vi "Init.vi"(7 "I2C #":T1=-1, 8 "error in (no error)":errorcluster, 10 "Session In":refnum<class "Session.lvclass">) -> (0 "error out":errorcluster, 3 "Grove Temperature Humidity Sensor DH20 Out":refnum<class "Grove Temperature Humidity Sensor DH20.lvclass">)   [LabVIEW 2020, in "CTI-Peripheral.lvlib" / "Grove Temperature Humidity Sensor DH20.lvclass"]
uses:
  Grove Temperature Humidity Sensor DH20.lvclass
  CTI/Session/Session.lvclass
  CTI/I2C Number.ctl
  CTI/I2C Address.ctl
  CTI/I2C Connection/I2C Connection.lvclass/I2C Connection.ctl
  Grove Temperature Humidity Sensor DH20.lvclass/Grove Temperature Humidity Sensor DH20.ctl
  CTI/I2C Connection/I2C Connection.lvclass
  CTI/CTI.lvlib
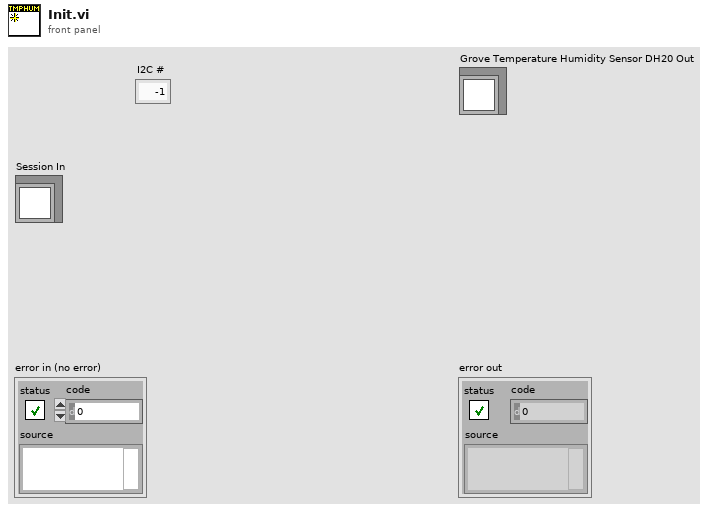
[diagram p1: front panel]
types:
  T1 = typedef "CTI.lvlib/I2C Number.ctl" = i8
  T2 = typedef "CTI.lvlib/I2C Address.ctl" = u8
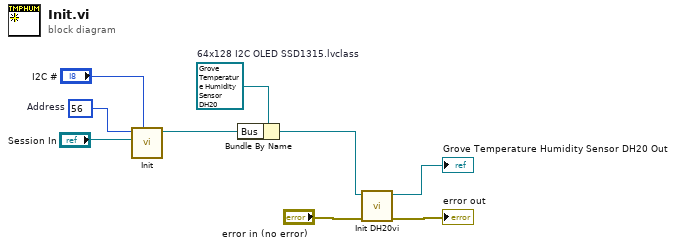
[diagram p0: block diagram]
diagram:
  w5 = refnum<class "Grove Temperature Humidity Sensor DH20.lvclass"> refnum  # 64x128 I2C OLED SSD1315.lvclass
  w6 = T2 56  # Address
  n1 = call "Init.vi"("I2C #"="I2C #", "Session"="Session In", "Address"=w6) -> ("I2C Connection"=w9:refnum<class "I2C Connection.lvclass">)  [unwired: 7 in, 1 out]
  n2 = Bundle By Name(cluster=w5, "Bus"=w9) -> (w4:refnum<class "Grove Temperature Humidity Sensor DH20.lvclass">)
  n3 = call "Init DH20vi.vi"("error in (no error)"="error in (no error)", "Grove Temperature Humidity Sensor DH20 in"=w4) -> ("error out"=→"error out":errorcluster, "6Grove Temperature Humidity Sensor DH20 out"=→"Grove Temperature Humidity Sensor DH20 Out":refnum<class "Grove Temperature Humidity Sensor DH20.lvclass">)  [unwired: 8 in]
